vi "Append JSON File.vi"(8 "error in (no error)":errorcluster, 10 "Path":path, 11 "Element in":variant) -> (0 "error out":errorcluster, 3 "Base Topology Variant out":variant)   [LabVIEW 2017]
uses:
  <vilib>/National Instruments/Variant JSON API/Variant JSON API.lvlib
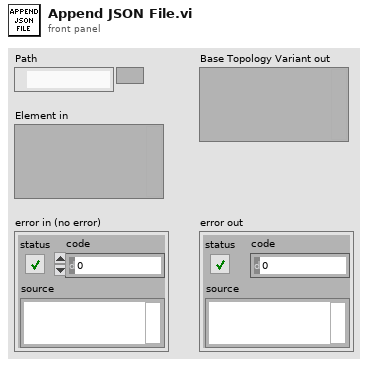
[diagram p1: front panel]
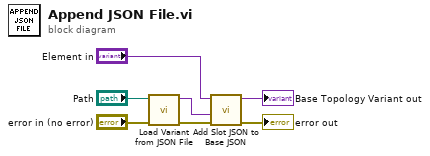
[diagram p0: block diagram]
diagram:
  n1 = call <vilib>:"Load Variant from JSON File.vi"("error in"="error in (no error)", "file path"="Path") -> ("error out"=w6:errorcluster, "Variant out"=w3:variant)  [unwired: 8 in]
  n2 = call "Add Slot JSON to Base JSON.vi"("error in (no error)"=w6, "Slot Topology Variant"=w3, "Base Topology Variant"="Element in") -> ("error out"=→"error out":errorcluster, "Base Topology Variant out"=→"Base Topology Variant out":variant)  [unwired: 7 in]
